vi "Get Protocol Type.vi"(8 "error in (no error)":errorcluster, 11 "protocol  in":refnum<class "Protocol Parent.lvclass">) -> (0 "error out":errorcluster, 2 "protocol type":T1=enum."AK RS-XXX", 3 "protocol out":refnum<class "Protocol Parent.lvclass">)   [LabVIEW 2020, in "Instrument Addon Scripting API.lvlib"]
doc: "Returns a protocol type Enum matching the protocol wired to the protocol in terminal."
uses:
  Instrument Addon Scripting API.lvlib
  Libraries Directory/Protocols.lvlibp/Protocol Parent/Protocol Parent.lvclass
  Libraries Directory/Protocols.lvlibp/Protocol Parent/Types/Protocol Type.ctl
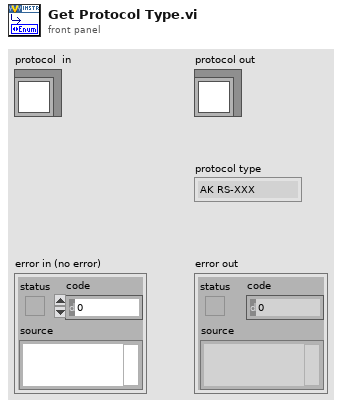
[diagram p1: front panel]
types:
  T1 = typedef "Protocols.lvlibp/Protocol Parent.lvclass/Protocol Type.ctl" = enum16{"RS-XXX", "AK RS-XXX", "VISA", "TCPIP", "AK TCPIP", "UDP", "GPIB ConvBox"}
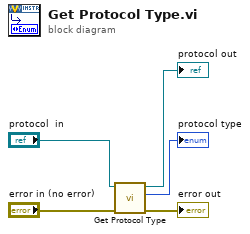
[diagram p0: block diagram]
diagram:
  n1 = call-dynamic "Get Protocol Type.vi"("error in (no error)"="error in (no error)", "protocol in"="protocol  in") -> ("error out"=→"error out":errorcluster, "protocol type"=→"protocol type":T1, "protocol out"=→"protocol out":refnum<class "Protocol Parent.lvclass">)  [unwired: 7 in]
